vi "SparseRandomProjection.vi"(8 "error in":errorcluster caption="entrée d'erreur", 11 "SparseRandomProjection":T1={"n_components"="auto", "density"="auto", "eps"=0.1, "dense_output"=FALSE, "random_state"=-1} {"random_state" min=-1; "eps" min=0.0}) -> (0 "error out":errorcluster caption="sortie d'erreur", 3 "SparseRandomProjection.lvclass":refnum<class "SparseRandomProjection.lvclass">)   [LabVIEW 2020]
doc: "Reduce dimensionality through sparse random projection\n\nSparse random matrix is an alternative to dense random projection matrix that guarantees similar embedding quality while being much more memory efficient and allowing faster computation of the projected data.\n\nIf we note s = 1 / density the components of the random matrix are drawn from :\n\n-sqrt(s) / sqrt(n_components) with probability 1 / 2s\n\n0 with probability 1 - 1 / s\n\n+sqrt(s) / sqrt(n_components) with probability 1 / 2s\n\n\nParameters : \n\n- n_components : int or ‘auto’, optional (default = ‘auto’)\nDimensionality of the target projection space.\n\nn_components can be automatically adjusted according to the number of samples in the dataset and the bound given by the Johnson-Lindenstrauss lemma. In that case the quality of the embedding is controlled by the eps parameter.\n\nIt should be noted that Johnson-Lindenstrauss lemma can yield very conservative estimated of the required number of components as it makes no assumption on the structure of the dataset.\n\n- density : float in range ]0, 1], optional (default=’auto’)\nRatio of non-zero component in the random projection matrix.\n\nIf density = ‘auto’, the value is set to the minimum density as recommended by Ping Li et al.: 1 / sqrt(n_features).\n\nUse density = 1 / 3.0 if you want to reproduce the results from Achlioptas, 2001.\n\n- eps : strictly positive float, optional=None=-1, (default=0.1)\nParameter to control the quality of the embedding according to the Johnson-Lindenstrauss lemma when n_components is set to ‘auto’.\n\nSmaller values lead to better embedding and higher number of dimensions (n_components) in the target projection space.\n\n- dense_output : boolean, optional (default=False)\nIf True, ensure that the output of the random projection is a dense numpy array even if the input and random projection matrix are both sparse. In practice, if the number of components is small the number of zero components in the projected data will be very small and it will be more CPU and memory efficient to use a dense representation.\n\nIf False, the projected data uses a sparse representation if the input is sparse.\n\n- random_state : int, RandomState instance or None, optional (default=None=-1)\nControls the pseudo random number generator used to generate the projection matrix at fit time. Pass an int for reproducible output across multiple function calls.\n\n\n\nMethods :\n\n- Fit : Generate a sparse random projection matrix\n\nParameters : X : numpy array or scipy.sparse of shape [n_samples, n_features]\n Training set : only the shape is used to find optimal random matrix dimensions based on the theory referenced in the afore mentioned papers.\n y : Ignored\n\n- Fit Transform : Fit to data, then transform it. Fits transformer to X and y with optional parameters fit_params and returns a transformed version of X.\n\nParameters : X : {array-like, sparse matrix, dataframe} of shape (n_samples, n_features)\n y : ndarray of shape (n_samples,), default=None\n Target values.\n\nReturns : X_new : ndarray array of shape (n_samples, n_features_new)\n Transformed array.\n\n\n- Transform : Project the data by using matrix product with the random matrix\n\nParameters : X : numpy array or scipy.sparse of shape [n_samples, n_features]\nThe input data to project into a smaller dimensional space.\n\nReturns : X_new : numpy array or scipy sparse of shape [n_samples, n_components]\nProjected array."
uses:
  SparseRandomProjection.lvclass
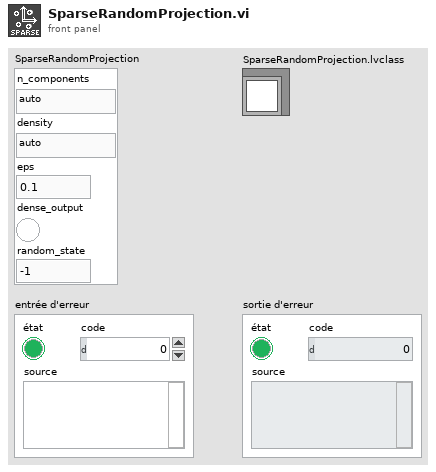
[diagram p1: front panel]
types:
  T1 = cluster{"n_components":string, "density":string, "eps":dbl, "dense_output":bool, "random_state":i32}
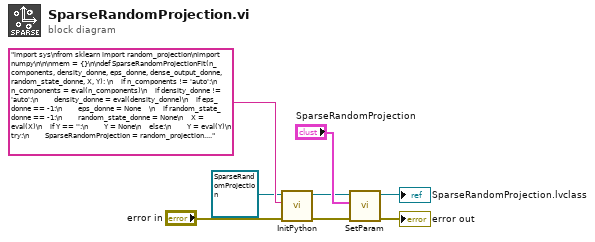
[diagram p0: block diagram]
diagram:
  n1 = call-dynamic "InitPython.vi"("error in (no error)"="error in", "Python Instruction"="import sys\nfrom sklearn import random_projection\nimport numpy\n\n\nmem = {}\n\ndef SparseRandomProjectionFit(n_components, density_donne, eps_donne, dense_output_donne, random_state_donne, X, Y): \n    if n_components != 'auto':\n        n_components = eval(n_components)\n    if density_donne != 'auto':\n        density_donne = eval(density_donne)\n    if eps_donne == -1:\n        eps_donne = None    \n    if random_state_donne == -1:\n        random_state_donne = None\n    X = eval(X)\n    if Y == '':\n        Y = None\n    else:\n        Y = eval(Y)\n    try:\n        SparseRandomProjection = random_projection.SparseRandomProjection(n_components, density = density_donne, eps = eps_donne , dense_output = dense_output_donne, random_state = random_state_donne).fit(X, Y)\n        mem['FitSparseRandomProjection'] = SparseRandomProjection\n        return str('OK')\n    except:\n        erreur = sys.exc_info()\n        typerr = u\"%s\" % (erreur[0])\n        typerr = typerr[typerr.find(\"'\")+1:typerr.rfind(\"'\")]\n        msgerr = u\"%s\" % (erreur[1])\n        message = str('/!\\\\ {0} : {1}'. format(typerr,msgerr))\n        return message \n\ndef SparseRandomProjectionFitTransform(n_components, density_donne, eps_donne, dense_output_donne, random_state_donne, X, Y):\n    if n_components != 'auto':\n        n_components = eval(n_components)\n    if density_donne != 'auto':\n        density_donne = eval(density_donne)\n    if eps_donne == -1:\n        eps_donne = None    \n    if random_state_donne == -1:\n        random_state_donne = None\n    X = eval(X)\n    if Y == '':\n        Y = None\n    else:\n        Y = eval(Y)\n    try:\n        SparseRandomProjection = random_projection.SparseRandomProjection(n_components, density = density_donne, eps = eps_donne , dense_output = dense_output_donne, random_state = random_state_donne).fit_transform(X, Y)\n        dtype = type(SparseRandomProjection)\n        if dtype == numpy.ndarray:\n            SparseRandomProjection = SparseRandomProjection.tolist()\n            return str(SparseRandomProjection)\n        else:\n            Mat = SparseRandomProjection.tocoo()\n            return str(list(zip(Mat.row, Mat.col, Mat.data)))\n    except:\n        erreur = sys.exc_info()\n        typerr = u\"%s\" % (erreur[0])\n        typerr = typerr[typerr.find(\"'\")+1:typerr.rfind(\"'\")]\n        msgerr = u\"%s\" % (erreur[1])\n        message = str('/!\\\\ {0} : {1}'. format(typerr,msgerr))\n        return message \n    \n\ndef SparseRandomProjectionTransform(n_components, density_donne, eps_donne, dense_output_donne, random_state_donne, X, Y):\n    if n_components != 'auto':\n        n_components = eval(n_components)\n    if density_donne != 'auto':\n        density_donne = eval(density_donne)\n    if eps_donne == -1:\n        eps_donne = None    \n    if random_state_donne == -1:\n        random_state_donne = None\n    X = eval(X)\n    if Y == '':\n        Y = None\n    else:\n        Y = eval(Y)\n    try:\n        SparseRandomProjection = mem['FitSparseRandomProjection'].transform(X, Y)\n        dtype = type(SparseRandomProjection)\n        if dtype == numpy.ndarray:\n            SparseRandomProjection = SparseRandomProjection.tolist()\n            return str(SparseRandomProjection)\n        else:\n            Mat = SparseRandomProjection.tocoo()\n            return str(list(zip(Mat.row, Mat.col, Mat.data)))\n    except:\n        erreur = sys.exc_info()\n        typerr = u\"%s\" % (erreur[0])\n        typerr = typerr[typerr.find(\"'\")+1:typerr.rfind(\"'\")]\n        msgerr = u\"%s\" % (erreur[1])\n        message = str('/!\\\\ {0} : {1}'. format(typerr,msgerr))\n        return message", "Scikit-learn en entrée"=refnum<class "SparseRandomProjection.lvclass"> refnum ("SparseRandomProjection.lvclass")) -> ("error out"=w6:errorcluster, "Scikit-learn en sortie"=w1:refnum<class "SparseRandomProjection.lvclass">)  [unwired: 7 in]
  n2 = call-dynamic "SetParam.vi"("error in (no error)"=w6, "SparseRandomProjection"="SparseRandomProjection", "SparseRandomProjection.lvclass"=w1) -> ("error out"=→"error out":errorcluster, "SparseRandomProjection.lvclass"=→"SparseRandomProjection.lvclass":refnum<class "SparseRandomProjection.lvclass">)  [unwired: 7 in]
